vi "ROI group-Get POI on sel plane only.vi"() -> (2 "POI on selected plane":dbl[][](array[numeric]))   [LabVIEW 2017]
uses:
  Typedefs/Get-Set-Clear Control.ctl
  Global variables/gl_Functional Imaging-Global variables.vi
panel:
  out "Norm. coord. of selected plane":dbl
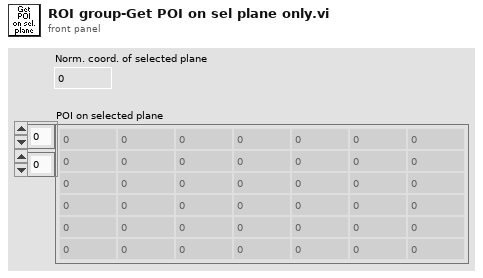
[diagram p1: front panel]
types:
  T1 = typedef "Get-Set-Clear Control.ctl" = enum16{"Get", "Set", "Clear"}
  T2 = typedef "Functional Imging UI Refs.ctl" = cluster{"Menu ref":refnum<k9>, "Image control":refnum<vi>, "VI ref":refnum<vi>, "XGrapher":refnum<vi>, "Smoothing":refnum<vi>, "POI Averaging":refnum<vi>, "Normalize":refnum<vi>, "POI data points in each trial":refnum<vi>, "Channel":refnum<vi>, "Experiment data folder path":refnum<vi>, "[ROI vis]":refnum<vi>, "[Groups] visbl":T3, "Group Name":refnum<vi>, "POI index":refnum<vi>, "Trial No.":refnum<vi>, "Intensity Zoom":refnum<vi>, "Trial Cursor Enabled":refnum<vi>, "Number of Trials (ind 1)":refnum<vi>, "Number of Trials (ind 2)":refnum<vi>, "MiniScans Available":refnum<vi>, "POI Available":refnum<vi>, "Defer graph updates":refnum<vi>, "Waveform selector":refnum<vi>, "#of selected POI":refnum<vi>, "#of selected MiniScans":refnum<vi>, "#of selected groups":refnum<vi>, "Max Z-Projection":refnum<vi>, "Z-Plane Selector":refnum<vi>, "Index of miniscan point to visualise":refnum<vi>, "ROI vis. mode":refnum<vi>, "Total # of points":refnum<vi>, "Index of group clicked on":refnum<vi>, "Pane 1":refnum<vi>, "Pane 2":refnum<vi>, "Pane 3":refnum<vi>, "Pane 4":refnum<vi>, "Pane 5":refnum<vi>, "Pane 6":refnum<vi>, "Deselect all ROI":refnum<vi>, "Deselect all groups":refnum<vi>}
  T3 = typedef "Groups array referecne.ctl" = refnum<vi>
  T4 = typedef "Functional Parameters Cluster.ctl" = cluster{"ROI data":dbl[][], "ROI format version":i32, "Norm ROI data":dbl[][], "Norm. ROI format version":i32, "Z norm":dbl[], "Z norm format version":i32}
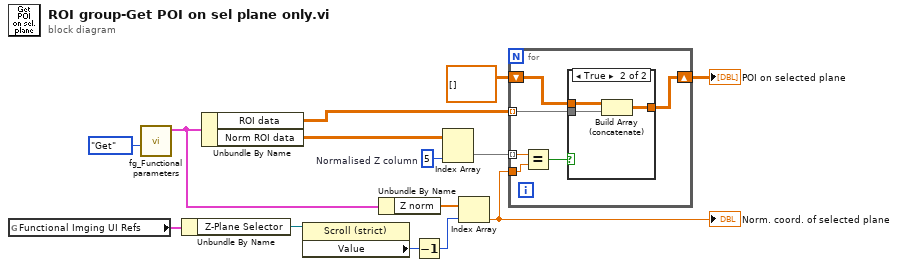
[diagram p0: block diagram]
diagram:
  w12 = 5  # Normalised Z column
  n1 = global read "gl_Functional Imaging-Global variables.vi" "Functional Imging UI Refs"() -> (w6:T2)
  n2 = call "fg_Functional parameters.vi"("Function"=Get-Set-Clear_Control."Get") -> ("Functional Parameters"=w3:T4)  [unwired: 7 in, 3 out]
  n3 = Unbundle By Name(w6) -> ("Z-Plane Selector"=w9:refnum<vi>)
  n4 = Unbundle By Name(w3) -> ("ROI data"=w1:dbl[][], "Norm ROI data"=w2:dbl[][])
  n5 = property class="Scroll (strict)"(reference=w9) -> ("Value"=w10:i32)  [unwired: 1 in, 2 out]
  n6 = Unbundle By Name(w3) -> ("Z norm"=w4:dbl[])
  n7 = Decrement(x=w10) -> (x-1=w7:i32)
  n8 = Index Array(array=w2, index (col)=w12) -> (element=w8:dbl[])  [unwired: 1 in]
  n9 = Index Array(array=w4, index=w7) -> (element=w11:dbl)
  "Norm. coord. of selected plane" <- w11
  n10 = for {
    tunnel: w8 -> [w20] mode=indexing
    tunnel: w11 -> [w19]
    tunnel: w1 -> [w17] mode=indexing
    shift-right: [w16] -> w14
    shift-left: dbl[][] [] -> [w15]
    n11 = Equal?(x=w20, y=w19) -> (x = y?=w18:bool)
    n12 = case shown="True" w18 {
      tunnel: w17 -> [_ w24]
      tunnel: [w21 w23] -> w16
      tunnel: w15 -> [w21 w22]
      frame False {
      }
      frame True {
        n13 = Build Array (concatenate)(w22, w24) -> (w23:dbl[][])
      }
    }
  }
  "POI on selected plane" <- w14
